vi "TCP_M 클라02.vi"() -> ()   [LabVIEW 2018]
panel:
  in  "종료시 문자열":string
  out "에러 출력":errorcluster
  out "웨이브폼 차트":i32(graph)
  in  "정지":bool
  in  "주소":string
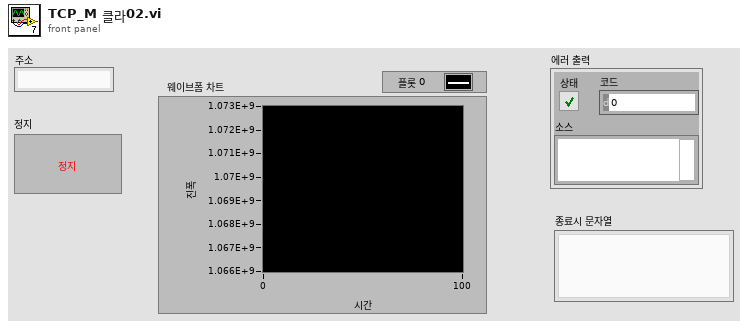
[diagram p1: front panel]
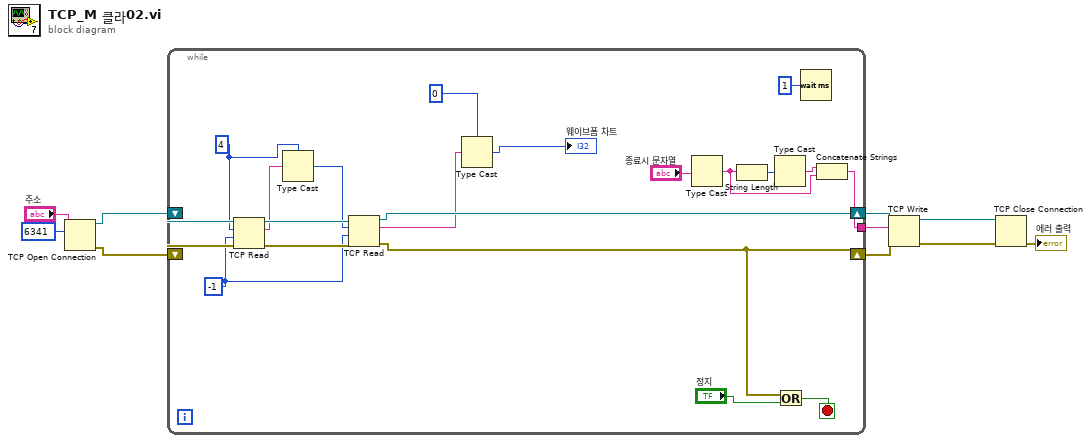
[diagram p0: block diagram]
diagram:
  n1 = TCP Open Connection(address="주소", remote port or service name=u16 6341 ("원격 포트 또는 서비스 이름")) -> (connection ID=w10:refnum<k5>, error out=w9:errorcluster)  [unwired: 3 in]
  n2 = while {
    shift-right: [w24] -> w3
    shift-left: w10 -> [w26]
    shift-right: [w28] -> w2
    shift-left: w9 -> [w31]
    tunnel: [w12] -> w1
    stop <- w27 stop-if-true
    w20 = -1 ("타임아웃 ms (25000)")
    w22 = 4 ("읽을 바이트")
    n3 = TCP Read(connection ID=w26, bytes to read=w22, error in (no error)=w31, 9:w20) -> (connection ID out=w25:refnum<k5>, data out=w23:string, error out=w30:errorcluster)  [unwired: 1 in]
    n4 = Type Cast(type=w22, x=w23) -> (*(type *) &x=w21:i32)
    n5 = TCP Read(connection ID=w25, bytes to read=w21, error in (no error)=w30, 9:w20) -> (connection ID out=w24:refnum<k5>, data out=w19:string, error out=w28:errorcluster)  [unwired: 1 in]
    n6 = Type Cast(type=0, x=w19) -> (*(type *) &x=→"웨이브폼 차트":i32)
    n7 = Type Cast(x="종료시 문자열") -> (*(type *) &x=w15:string)  [unwired: 1 in]
    n8 = String Length(string=w15) -> (length=w14:i32)
    n9 = Type Cast(x=w14) -> (*(type *) &x=w16:string)  [unwired: 1 in]
    n10 = Or(x=w28, y="정지") -> (x .or. y?=w27:bool)
    n11 = Wait (ms)(milliseconds to wait=u32 1 ("대기 시간 (ms)")) -> ()  [unwired: 1 out]
    n12 = Concatenate Strings(w16, w15) -> (w12:string)
  }
  n13 = TCP Write(connection ID=w3, data in=w1, error in (no error)=w2) -> (connection ID out=w5:refnum<k5>, error out=w6:errorcluster)  [unwired: 1 in, 1 out]
  n14 = TCP Close Connection(connection ID=w5, error in (no error)=w6) -> (error out=→"에러 출력":errorcluster)  [unwired: 1 in, 1 out]
